vi "Get Configuration.vi"(0 "gRPCid":T1, 5 "Service Class":string, 11 "error in (no error)":errorcluster) -> (4 "Measurement Config":refnum<vi>, 6 "Measurement Results":refnum<vi>, 15 "error out":errorcluster)   [LabVIEW 2021, in "Measurement Client.lvlib"]
uses:
  Measurement Client.lvlib
  <vilib>/gRPC/Generated APIs/ni/measurementlink/discovery/v1/ni.measurementlink.discovery.v1.api.lvlib
  Runtime/Clients/Measurement Service Client V2/Measurement Service Client V2.lvlib
  <vilib>/gRPC/Generated APIs/ni/measurementlink/discovery/v1/RPC Messages/ni_measurementlink_discovery_v1_ResolveServiceRequest.ctl
  <vilib>/gRPC/LabVIEW gRPC Library/Shared/grpcId.ctl
  <vilib>/gRPC/LabVIEW gRPC Library/grpc-lvsupport-release.lvlib
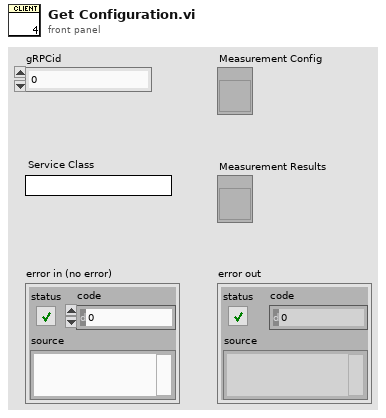
[diagram p1: front panel]
types:
  T1 = typedef "grpc-lvsupport-release.lvlib/grpcId.ctl" = u64
  T2 = typedef "ni.measurementlink.discovery.v1.api.lvlib/ni_measurementlink_discovery_v1_ResolveServiceRequest.ctl" = cluster{"provided_interface":string, "service_class":string}
  T3 = typedef "ni.measurementlink.discovery.v1.api.lvlib/ni_measurementlink_discovery_v1_ServiceLocation.ctl" = cluster{"location":string, "insecure_port":string, "ssl_authenticated_port":string}
  T4 = typedef "Measurement Service Client V2.lvlib/ni_measurementlink_measurement_v2_GetMetadataResponse.ctl" = cluster{"measurement_details":T5, "measurement_signature":T6, "user_interface_details":T13[]}
  T5 = typedef "Measurement Service Client V2.lvlib/ni_measurementlink_measurement_v2_MeasurementDetails.ctl" = cluster{"display_name":string, "version":string}
  T6 = typedef "Measurement Service Client V2.lvlib/ni_measurementlink_measurement_v2_MeasurementSignature.ctl" = cluster{"configuration_parameters_message_type":string, "configuration_parameters":T7[], "configuration_defaults":T10, "outputs_message_type":string, "outputs":T11[]}
  T7 = typedef "Measurement Service Client V2.lvlib/ni_measurementlink_measurement_v2_ConfigurationParameter.ctl" = cluster{"field_number":i32, "type":T8, "name":string, "repeated":bool, "annotations":T9[], "message_type":string}
  T8 = typedef "Measurement Service Client V2.lvlib/google_protobuf_Field_Kind.ctl" = enum32{"TYPE_UNKNOWN", "TYPE_DOUBLE", "TYPE_FLOAT", "TYPE_INT64", "TYPE_UINT64", "TYPE_INT32", "TYPE_FIXED64", "TYPE_FIXED32", "TYPE_BOOL", "TYPE_STRING", "TYPE_GROUP", "TYPE_MESSAGE", "TYPE_BYTES", "TYPE_UINT32", "TYPE_ENUM", "TYPE_SFIXED32", "TYPE_SFIXED64", "TYPE_SINT32", "TYPE_SINT64"}
  T9 = typedef "Measurement Service Client V2.lvlib/ni_measurementlink_measurement_v2_ConfigurationParameter_AnnotationsEntry.ctl" = cluster{"key":string, "value":string}
  T10 = typedef "Measurement Service Client V2.lvlib/google_protobuf_Any.ctl" = cluster{"type_url":string, "value":u8[]}
  T11 = typedef "Measurement Service Client V2.lvlib/ni_measurementlink_measurement_v2_Output.ctl" = cluster{"field_number":i32, "type":T8, "name":string, "repeated":bool, "annotations":T12[], "message_type":string}
  T12 = typedef "Measurement Service Client V2.lvlib/ni_measurementlink_measurement_v2_Output_AnnotationsEntry.ctl" = cluster{"key":string, "value":string}
  T13 = typedef "Measurement Service Client V2.lvlib/ni_measurementlink_measurement_v2_UserInterfaceDetails.ctl" = cluster{"file_url":string}
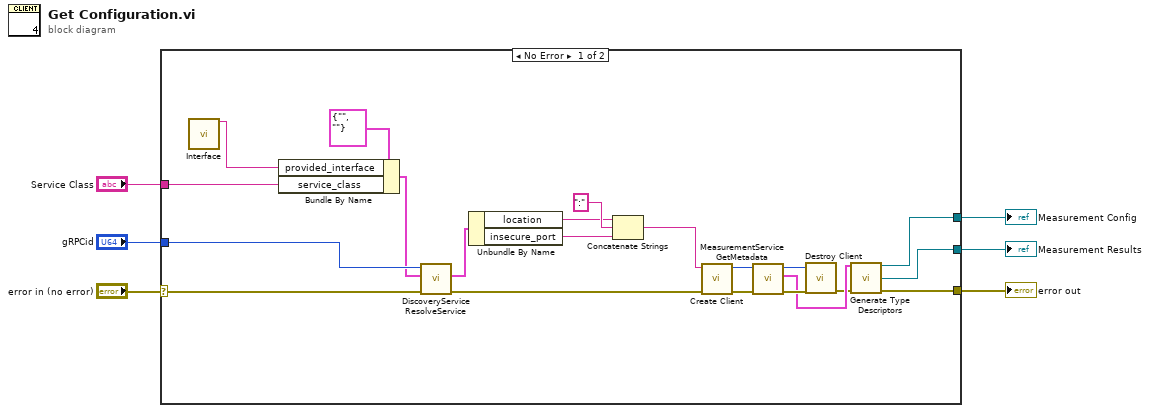
[diagram p0: block diagram]
diagram:
  n1 = case shown="No Error" "error in (no error)" {
    selector: "error in (no error)" -> [w8 w28]
    tunnel: "gRPCid" -> [w27 _]
    tunnel: [w23 _] -> w5
    tunnel: [w22 _] -> w4
    tunnel: [w9 w28] -> w3
    tunnel: "Service Class" -> [w7 _]
    frame No Error {
      n2 = call "Interface.vi"() -> ("Interface"=w24:string)  [unwired: 15 in]
      n3 = Bundle By Name(cluster=T2 {"provided_interface"="", "service_class"=""} ("Request Data"), "provided_interface"=w24, "service_class"=w7) -> (w26:T2)
      n4 = call <vilib>:"DiscoveryService ResolveService.vi"("error in"=w8, "Request Data"=w26, "gRPC ID"=w27) -> ("error out"=w12:errorcluster, "Response Data"=w18:T3)  [unwired: 6 in, 1 out]
      n5 = Unbundle By Name(w18) -> ("location"=w19:string, "insecure_port"=w21:string)
      n6 = Concatenate Strings(w19, ":" ("string"), w21) -> (w13:string)
      n7 = call "Create Client.vi"("error in"=w12, "address"=w13) -> ("error out"=w14:errorcluster, "gRPC ID Out"=w15:T1)  [unwired: 8 in]
      n8 = call "MeasurementService GetMetadata.vi"("error in"=w14, "gRPC ID"=w15) -> ("error out"=w16:errorcluster, "Response Data"=w11:T4, "gRPC ID out"=w17:T1)  [unwired: 7 in]
      n9 = call "Destroy Client.vi"("error in"=w16, "gRPC ID"=w17) -> ("error out"=w10:errorcluster)  [unwired: 9 in]
      n10 = call "Generate Type Descriptors.vi"("Measurement Metadata"=w11, "error in (no error)"=w10) -> ("Configs Type"=w22:refnum<vi>, "Outputs Type"=w23:refnum<vi>, "error out"=w9:errorcluster)  [unwired: 9 in, 2 out]
    }
    frame Error {
    }
  }
  "Measurement Results" <- w5
  "Measurement Config" <- w4
  "error out" <- w3
